vi "Customize VI Window.vi"() -> ()   [LabVIEW 2010]
doc: "This VI demonstrates VI Server methods and properties: Show Menu Bar, Show Title Bar, VI Transparency, and Centering the VI."
panel:
  in  "Center":bool
  in  "stop":bool
  in  "Make VI Transparent?":bool
  in  "Show Title Bar?":bool
  in  "Show Menu Bar?":bool
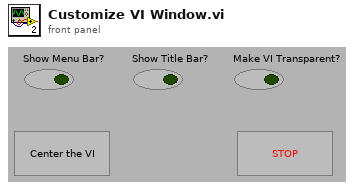
[diagram p1: front panel]
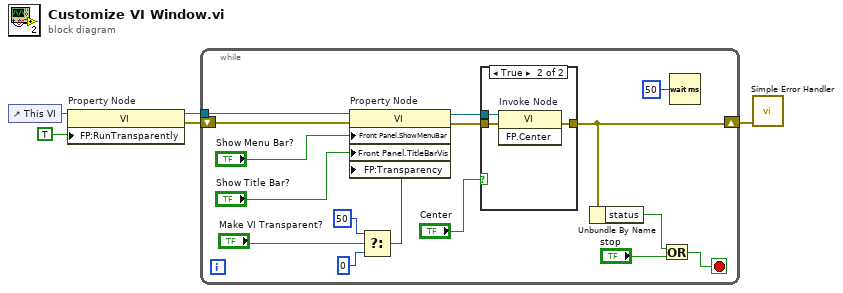
[diagram p0: block diagram]
diagram:
  n1 = control-ref of="This VI"() -> (w5:refnum<vi>)
  n2 = property on="Property Node" class="VI"(reference=w5, "FP:RunTransparently"=TRUE ("Front Panel Window:Run VI Transparently")) -> (reference out=w3:refnum<vi>, error out=w2:errorcluster)  [unwired: 1 in]
  n3 = while {
    tunnel: w3 -> [w21]
    shift-right: [w9] -> w1
    shift-left: w2 -> [w20]
    stop <- w10 stop-if-true
    n4 = Select(t=50, s="Make VI Transparent?", f=0) -> (s? t:f=w14:i32)
    n5 = property on="Property Node" class="VI"(reference=w21, error in=w20, "Front Panel.ShowMenuBar"="Show Menu Bar?", "Front Panel.TitleBarVis"="Show Title Bar?", "FP:Transparency"=w14) -> (reference out=w11:refnum<vi>, error out=w12:errorcluster)
    n6 = case shown="True" "Center" {
      tunnel: w12 -> [w22 w25]
      tunnel: [w22 w24] -> w9
      tunnel: w11 -> [_ w23]
      frame False {
      }
      frame True {
        n7 = invoke on="Invoke Node" class="VI" method="FP.Center"(reference=w23, error in=w25) -> (error out=w24:errorcluster)  [unwired: 1 in, 2 out]
      }
    }
    n8 = Unbundle By Name(w9) -> ("status"=w8:bool)
    n9 = Or(x=w8, y="stop") -> (x .or. y?=w10:bool)
    n10 = Wait (ms)(milliseconds to wait=u32 50) -> ()  [unwired: 1 out]
  }
  n11 = call <vilib>:"Simple Error Handler.vi"("error in (no error)"=w1) -> ()  [unwired: 4 in, 5 out]
